vi "IO@AddVirtualIO__Parameter.vi"(1 "ParamterIn":string) -> (0 "ParamterOut":string)   [LabVIEW 2019]
panel:
  in  "ON/OFF":string(combo)="On"
  in  "PortSelect":string(combo)
  in  "Confirm":bool
  # "IO@AddVirtualIO $IOName,On/Off\nIO@AddVirtualIO $IOName,$Logic"
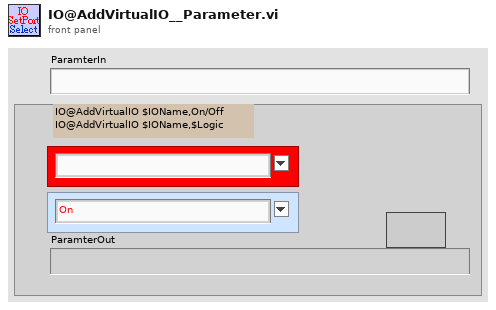
[diagram p1: front panel]
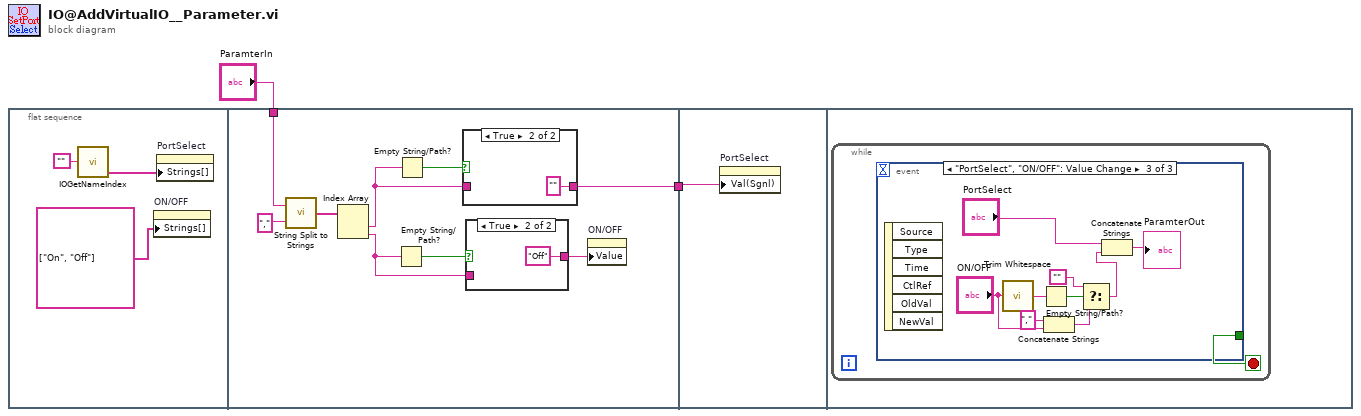
[diagram p0: block diagram]
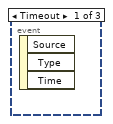
[diagram p4: hidden frame]
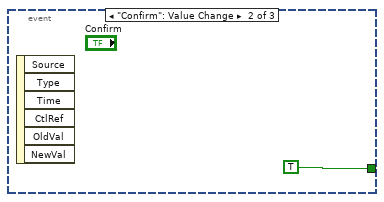
[diagram p5: hidden frame]
diagram:
  n1 = flat-sequence {
    tunnel: "ParamterIn" -> [w13]
    tunnel: [w6] -> w1
    tunnel: w1 -> [w19]
    frame #0 {
      n2 = call "IOGetNameIndex.vi"("PortName"="") -> ("PortNameList Out"=w4:string[])  [unwired: 3 in, 1 out]
      n3 = property on="ON/OFF" class="CmbBox"("Strings[]"=string[] ["On", "Off"] ("Strings []")) -> ()  [unwired: 2 in, 2 out]
      n4 = property on="PortSelect" class="CmbBox"("Strings[]"=w4) -> ()  [unwired: 2 in, 2 out]
    }
    frame #1 {
      n5 = call "String Split to Strings.vi"("search string/char (-)"=",", "String"=w13) -> ("Array"=w12:string[])
      n6 = Index Array(array=w12) -> (element #1=w10:string, element #2=w8:string)  [unwired: 2 in]
      n7 = Empty String/Path?(string/path=w8) -> (empty?=w9:bool)
      n8 = Empty String/Path?(string/path=w10) -> (empty?=w11:bool)
      n9 = case shown="True" w11 {
        tunnel: w10 -> [w17 _]
        tunnel: [w17 ""] -> w6
        frame False {
        }
        frame True {
        }
      }
      n10 = case shown="True" w9 {
        tunnel: w8 -> [w15 _]
        tunnel: [w15 "Off"] -> w7
        frame False {
        }
        frame True {
        }
      }
      n11 = property on="ON/OFF" class="CmbBox"("Value"=w7) -> ()  [unwired: 2 in, 2 out]
    }
    frame #2 {
      n12 = property on="PortSelect" class="CmbBox"("Val(Sgnl)"=w19) -> ()  [unwired: 2 in, 2 out]
    }
    frame #3 {
      n13 = while {
        stop <- w20 stop-if-true
        n14 = event shown="[2] \"PortSelect\", \"ON/OFF\": Value Change" {
          selector: _ -> [_ _ _]
          dyn-events: _ -> [_ _ _]
          timeout: _ -> [_ _ _]
          tunnel: [_ TRUE _] -> w20
          event Timeout {
            n15 = event-data() -> ()  [unwired: 1 in, 3 out]
          }
          event "Confirm": Value Change {
            n16 = event-data() -> ()  [unwired: 1 in, 6 out]
          }
          event "PortSelect", "ON/OFF": Value Change {
            n17 = event-data() -> ()  [unwired: 1 in, 6 out]
            n18 = call <vilib>:"Trim Whitespace.vi"("string"="ON/OFF") -> ("trimmed string"=w28:string)  [unwired: 1 in]
            n19 = Empty String/Path?(string/path=w28) -> (empty?=w27:bool)
            n20 = Concatenate Strings("," ("string"), "ON/OFF") -> (w25:string)
            n21 = Select(t="", s=w27, f=w25) -> (s? t:f=w22:string)
            n22 = Concatenate Strings("PortSelect", w22) -> (→"ParamterOut":string)
          }
        }
      }
    }
  }
